vi "Detect rising edge.vi"(10 "signal":bool=TRUE) -> (2 "edge detected":bool)   [LabVIEW 2020]
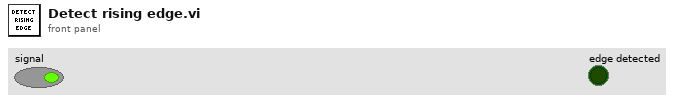
[diagram p1: front panel]
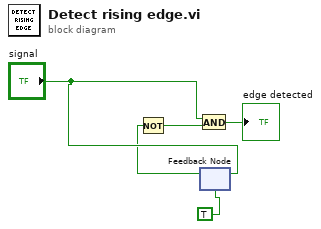
[diagram p0: block diagram]
diagram:
  n1 = feedback-in #1("signal") -> ()
  n2 = feedback #1(TRUE ("signal")) -> (w2:bool)
  n3 = Not(x=w2) -> (.not. x?=w3:bool)
  n4 = And(x="signal", y=w3) -> (x .and. y?=→"edge detected":bool)
